vi "PQclear.vi"(8 "error in":errorcluster, 10 "res":u64, 11 "conn":u64) -> (0 "error out":errorcluster, 3 "conn_out":u64)   [LabVIEW 2019, in "libpqutility64.lvlib"]
uses:
  libpqutility64.lvlib
  libpqlv64/libpqlv64.lvlib
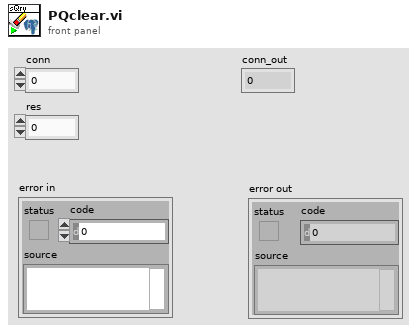
[diagram p1: front panel]
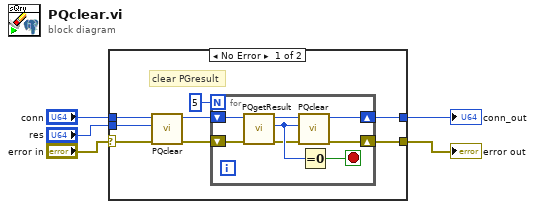
[diagram p0: block diagram]
diagram:
  n1 = case shown="No Error" "error in" {
    selector: "error in" -> [w7 w22]
    tunnel: "conn" -> [w8 w23]
    tunnel: [w11 w23] -> w3
    tunnel: [w6 w22] -> w2
    tunnel: "res" -> [w9 _]
    frame No Error {
      # "clear PGresult"
      n2 = call "PQclear.vi"("error in (no error)"=w7, "res"=w9, "conn"=w8) -> ("error out"=w10:errorcluster, "conn_out"=w12:u64)  [unwired: 7 in]
      n3 = for {
        N: 5 -> [_]
        shift-right: [w17] -> w11
        shift-left: w12 -> [w18]
        shift-right: [w14] -> w6
        shift-left: w10 -> [w16]
        stop <- w20 stop-if-true
        n4 = call "PQgetResult.vi"("error in (no error)"=w16, "conn"=w18) -> ("error out"=w15:errorcluster, "PGresult"=w19:u64, "conn_out"=w21:u64)  [unwired: 7 in]
        n5 = call "PQclear.vi"("error in (no error)"=w15, "res"=w19, "conn"=w21) -> ("error out"=w14:errorcluster, "conn_out"=w17:u64)  [unwired: 7 in]
        n6 = Equal To 0?(x=w19) -> (x = 0?=w20:bool)
      }
    }
    frame Error {
    }
  }
  "conn_out" <- w3
  "error out" <- w2
